vi "TGS.vi"(0 "System no.":i32=1 min=1 max=4 step=1, 2 "Trajectory ID":i32[](array[numeric]), 3 "Start all?":bool, 5 "error in":errorcluster) -> (19 "error out":errorcluster)   [LabVIEW 2020]
doc: "Start trajectories. For further details, see Trajectories for Motion Paths in the controller user manual.\n\nC-867, C-884:"
panel:
  # "Start trajectories."
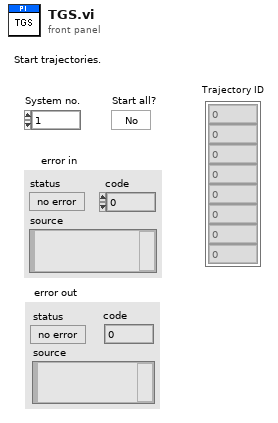
[diagram p1: front panel]
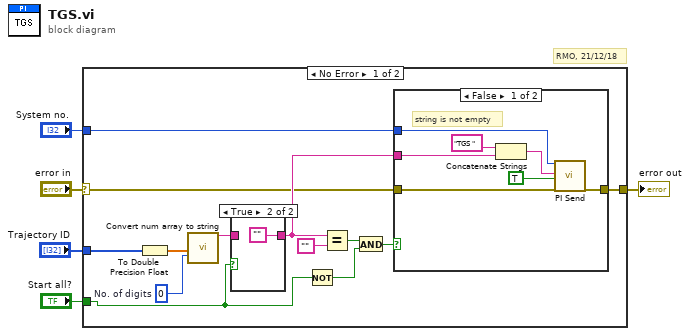
[diagram p0: block diagram]
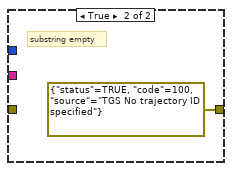
[diagram p3: hidden frame]
diagram:
  # "RMO, 21/12/18"
  n1 = case shown="No Error" "error in" {
    selector: "error in" -> [w6 w29]
    tunnel: [w18 w29] -> w5
    tunnel: "System no." -> [w17 _]
    tunnel: "Trajectory ID" -> [w10 _]
    tunnel: "Start all?" -> [w7 _]
    frame No Error {
      w16 = i16 0  # No. of digits
      n2 = To Double Precision Float(number=w10) -> (double precision float=w11:dbl[])
      n3 = call "Convert num array to string.vi"("Num. values"=w11, "No. of digits"=w16) -> ("Output string"=w9:string)  [unwired: 17 out]
      n4 = case shown="True" w7 {
        tunnel: w9 -> [w19 _]
        tunnel: [w19 "" ("y")] -> w8
        frame False {
        }
        frame True {
        }
      }
      n5 = Not(x=w7) -> (.not. x?=w12:bool)
      n6 = Equal?(x=w8, y="") -> (x = y?=w13:bool)
      n7 = And(x=w13, y=w12) -> (x .and. y?=w15:bool)
      n8 = case shown="False" w15 {
        tunnel: w8 -> [w26 _]
        tunnel: [w22 errorcluster {"status"=TRUE, "code"=100, "source"="TGS No trajectory ID specified"} ("error out")] -> w18
        tunnel: w6 -> [w23 _]
        tunnel: w17 -> [w21 _]
        frame False {
          # "string is not empty"
          n9 = Concatenate Strings("TGS ", w26) -> (w24:string)
          n10 = call "PI Send.vi"("System no."=w21, "String to send"=w24, "Attach termination char.?"=TRUE ("Attach Linefeed?"), "error in"=w23) -> ("error out"=w22:errorcluster)  [unwired: 2 in, 13 out]
        }
        frame True {
          # "substring empty"
        }
      }
    }
    frame Error {
    }
  }
  "error out" <- w5
